vi "Configure Measurement Delay.vi"(8 "error in (no error)":errorcluster, 9 "Edge Specific 2 (0)":i32, 10 "Edge Specific 1 (0)":i32, 11 "VISA resource name":refnum<visa-resource-name>) -> (0 "error out":errorcluster, 3 "VISA resource name out":refnum<visa-resource-name>)   [LabVIEW 2017, in "Agilent 6000 Series.lvlib"]
doc: "This VI configures the properties that control the measurement delay. These properties are specifies the edge 1 and edge 2."
uses:
  <instrlib>/Agilent 6000 Series/Agilent 6000 Series.lvlib
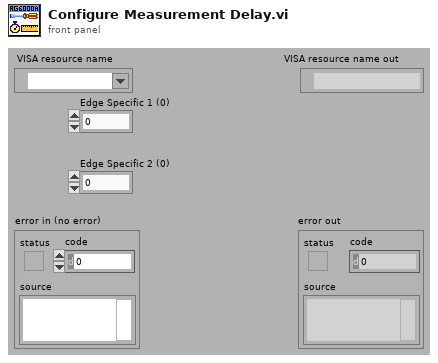
[diagram p1: front panel]
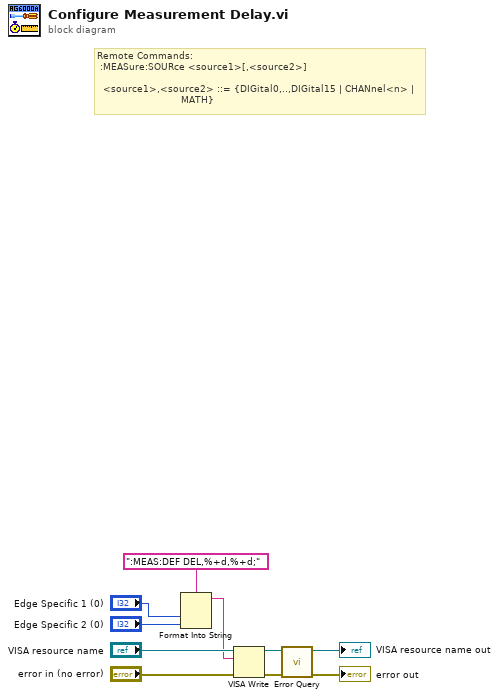
[diagram p0: block diagram]
diagram:
  # "Remote Commands:\n :MEASure:SOURce <source1>[,<source2>]\n\n  <source1>,<source2> ::= {DIGital0,..,DIGital15 | CHANnel<n> | \n                            MATH}"
  n1 = Format Into String(format string=":MEAS:DEF DEL,%+d,%+d;", "Edge Specific 1 (0)", "Edge Specific 2 (0)") -> (resulting string=w1:string)  [unwired: 2 in, 1 out]
  n2 = VISA Write(VISA resource name="VISA resource name", write buffer=w1, error in (no error)="error in (no error)") -> (VISA resource name out=w6:refnum<visa-resource-name>, error out=w5:errorcluster)  [unwired: 1 out]
  n3 = call <instrlib>:"Error Query.vi"("error in (no error)"=w5, "VISA resource name"=w6) -> ("error out"=→"error out":errorcluster, "VISA resource name out"=→"VISA resource name out":refnum<visa-resource-name>)  [unwired: 6 in, 2 out]
